vi "find channel.vi"(9 "settings id":string, 11 "DSFConfiguration in":refnum<class "DSFConfiguration.lvclass">) -> (2 "index":i32)   [LabVIEW 2017, in "DSFConfiguration.lvclass"]
uses:
  DSFConfiguration.lvclass
  DSFConfiguration.lvclass/DSFConfiguration.ctl
  DSFChannel/DSFChannel.lvclass/DSFChannel.ctl
  DSFChannel/DSFChannel.lvclass
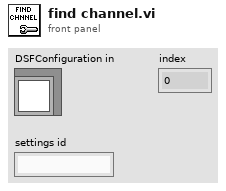
[diagram p1: front panel]
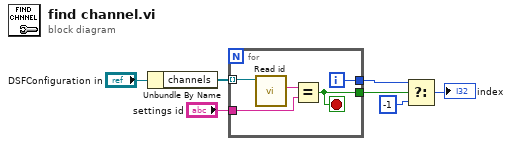
[diagram p0: block diagram]
diagram:
  n1 = Unbundle By Name("DSFConfiguration in") -> ("channels"=w7:refnum<class "DSFChannel.lvclass">[])
  n2 = for {
    tunnel: w7 -> [w12] mode=indexing
    tunnel: "settings id" -> [w10]
    tunnel: [w9] -> w2
    tunnel: [w8] -> w3
    i -> [w9]
    stop <- w8 stop-if-true
    n3 = call "Read id.vi"("DSFChannel in"=w12) -> ("id"=w11:string)  [unwired: 8 in, 2 out]
    n4 = Equal?(x=w11, y=w10) -> (x = y?=w8:bool)
  }
  n5 = Select(t=w2, s=w3, f=-1) -> (s? t:f=→"index":i32)
